vi "ValChange.vi"(6 "Value":string, 7 "Col Array Ref in":refnum<vi>, 8 "error in (no error)":errorcluster, 9 "Table CtlRef In":refnum<vi>, 10 "Cell Position":T1, 11 "MenuDisableCol in":refnum<class "MenuDisableCol.lvclass">) -> (0 "error out":errorcluster, 1 "Table CtlRef Out":refnum<vi>, 3 "MenuDisableCol out":refnum<class "MenuDisableCol.lvclass">)   [LabVIEW 2013, in "MenuDisableCol.lvclass"]
doc: "If a table cell value changes, calling this method will ensure the change is pushed down to any subsequent disabled cells.\nThis is read only w.r.t. column data (only for dynamic dispatch)."
uses:
  MenuDisableCol.lvclass
  <vilib>/Utility/miscctls.llb/LVRowAndColumnTypeDef.ctl
  MenuCol/MenuCol.lvclass
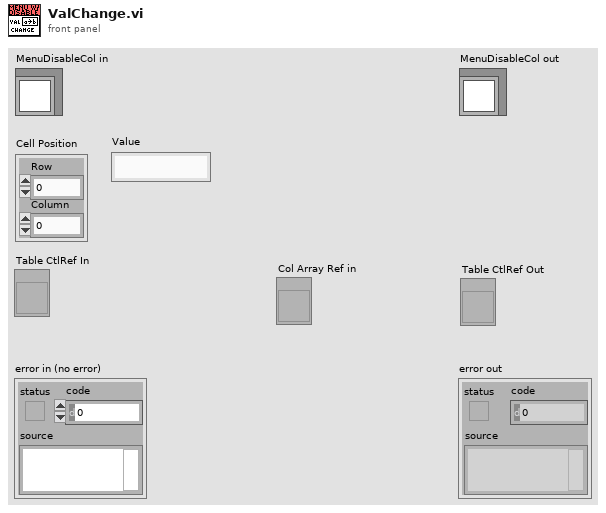
[diagram p1: front panel]
types:
  T1 = typedef "LVRowAndColumnTypeDef.ctl" = cluster{"Row":i32, "Column":i32}
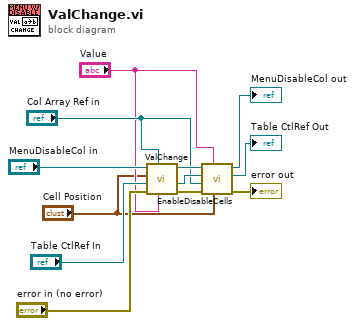
[diagram p0: block diagram]
diagram:
  n1 = call-parent "ValChange.vi"("Value"="Value", "Col Array Ref in"="Col Array Ref in", "error in (no error)"="error in (no error)", "Table CtlRef In"="Table CtlRef In", "Cell Position"="Cell Position", "MenuCol in"="MenuDisableCol in") -> ("error out"=w5:errorcluster, "Table CtlRef Out"=w8:refnum<vi>, "MenuCol out"=w9:refnum<class "MenuDisableCol.lvclass">)  [unwired: 3 in]
  n2 = call-dynamic "EnableDisableCells.vi"("Cell Position"="Cell Position", "Item Name or Tag"="Value", "error in (no error)"=w5, "Col Array Ref in"="Col Array Ref in", "Table CtlRef in"=w8, "MenuDisableCol in"=w9) -> ("error out"=→"error out":errorcluster, "Table CtlRef out"=→"Table CtlRef Out":refnum<vi>, "MenuDisableCol out"=→"MenuDisableCol out":refnum<class "MenuDisableCol.lvclass">)  [unwired: 2 in, 1 out]
